vi "Do Query.vi"(9 "Query Builder":refnum<class "Query Builder.lvclass">, 11 "Database in":refnum<class "SQLite.lvclass">) -> (0 "error out":errorcluster, 2 "Results":refnum<class "Result Row.lvclass">[](array[class]), 3 "Database out":refnum<class "SQLite.lvclass">)   [LabVIEW 2020, in "Conditum SQLite.lvlib" / "SQLite.lvclass"]
uses:
  SQLite.lvclass
  <vilib>/IlluminatedG/IG Conditum/Conditum/Query Builder/Query Builder.lvclass
  <vilib>/IlluminatedG/IG Conditum/Conditum/Result Row/Result Row.lvclass
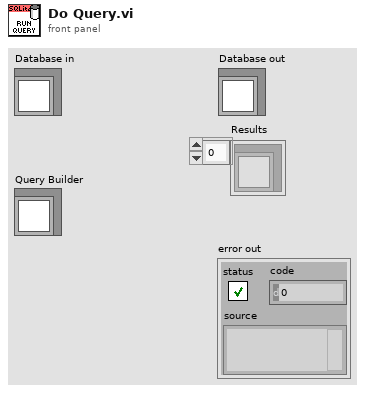
[diagram p1: front panel]
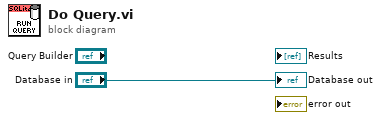
[diagram p0: block diagram]
diagram:
  "Database out" <- "Database in"
